vi "Handle Mouse Wheel.vi"(8 "error in (no error)":errorcluster, 10 "delta":i32, 11 "Array Refnum":refnum<vi>) -> (0 "error out":errorcluster, 3 "Array Refnum":refnum<vi>)   [LabVIEW 2017, in "UI Common.lvlib"]
uses:
  UI Common.lvlib
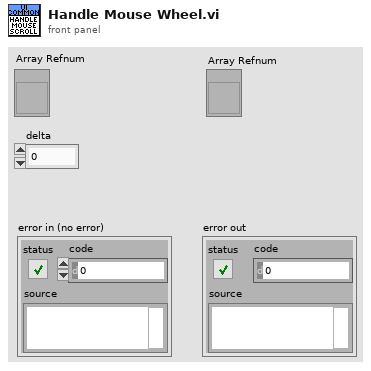
[diagram p1: front panel]
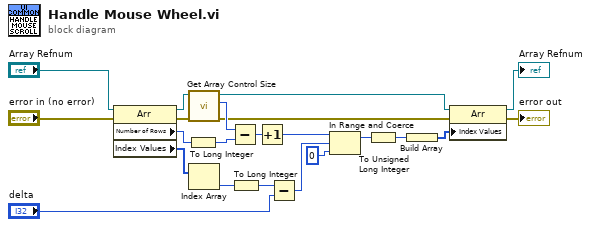
[diagram p0: block diagram]
diagram:
  n1 = property class="Arr"(reference="Array Refnum", error in="error in (no error)") -> (reference out=w19:refnum<vi>, error out=w18:errorcluster, "Number of Rows"=w5:u32, "Index Values"=w20:u32[])
  n2 = To Long Integer(number=w5) -> (32bit integer=w16:i32)
  n3 = call "Get Array Control Size.vi"("error in (no error)"=w18, "Array in"=w19) -> ("error out"=w9:errorcluster, "Size"=w17:i32, "Array out"=w10:refnum<vi>)  [unwired: 7 in]
  n4 = Index Array(array=w20) -> (element=w4:u32)  [unwired: 1 in]
  n5 = Subtract(x=w17, y=w16) -> (x-y=w15:i32)
  n6 = To Long Integer(number=w4) -> (32bit integer=w6:i32)
  n7 = Increment(x=w15) -> (x+1=w3:i32)
  n8 = Subtract(x=w6, y="delta") -> (x-y=w1:i32)
  n9 = In Range and Coerce(upper limit=w3, x=w1, lower limit=0) -> (coerced(x)=w13:i32)  [unwired: 1 out]
  n10 = To Unsigned Long Integer(number=w13) -> (unsigned 32bit integer=w12:u32)
  n11 = Build Array(w12) -> (w11:u32[])
  n12 = property class="Arr"(reference=w10, error in=w9, "Index Values"=w11) -> (reference out=→"Array Refnum":refnum<vi>, error out=→"error out":errorcluster)
